vi "timeOfDayFromSS1904.vi"() -> (0 "New Values In":string[][](array[string])=[["Test data5"]], 1 "New Chs In":string[](array[string])=["30-10-03:New:Channel new5"])   [LabVIEW 2022 SP3]
uses:
  Data plotting/subVIs/Plot_Values_Global.vi
panel:
  # "Using SS1/1/1904 on the X-axis, adds channels for Hour and Minute"
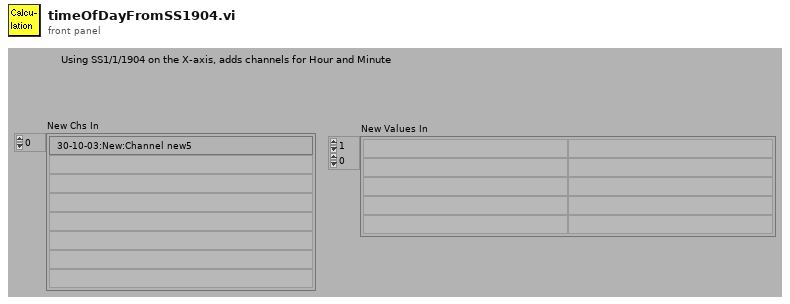
[diagram p1: front panel]
types:
  T1 = typedef "LVDateTimeRec.ctl" = cluster{"fractional second":dbl, "second":i32, "minute":i32, "hour":i32, "day of month":i32, "month":i32, "year":i32, "day of week":i32, "day of year":i32, "DST":i32}
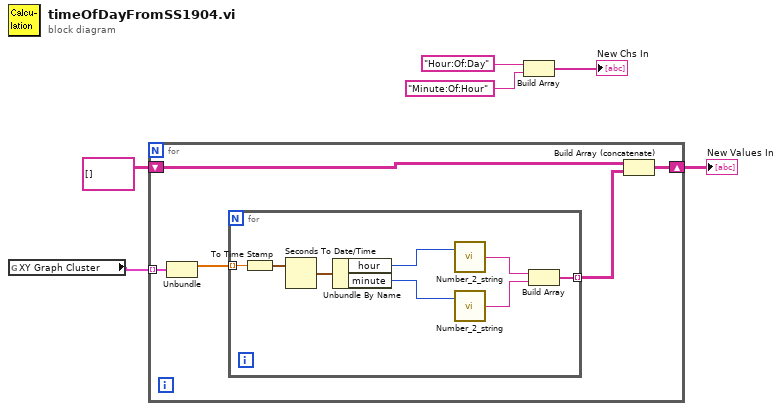
[diagram p0: block diagram]
diagram:
  n1 = global read "Plot_Values_Global.vi" "XY Graph Cluster"() -> (w2:cluster{dbl[], dbl[]}[])
  n2 = for {
    tunnel: w2 -> [w11] mode=indexing
    shift-right: [w9] -> w4
    shift-left: string[][] [] -> [w10]
    n3 = Unbundle(w11) -> (w7:dbl[])  [unwired: 1 out]
    n4 = for {
      tunnel: w7 -> [w17] mode=indexing
      tunnel: [w18] -> w8 mode=indexing
      n5 = To Time Stamp(1:w17) -> (0:w16:timestamp)
      n6 = Seconds To Date/Time(time stamp (now)=w16) -> (date time rec=w15:T1)  [unwired: 1 in]
      n7 = Unbundle By Name(w15) -> ("hour"=w14:i32, "minute"=w13:i32)
      n8 = call "Number_2_string.vi"("number"=w14) -> ("String"=w19:string)  [unwired: 1 in]
      n9 = call "Number_2_string.vi"("number"=w13) -> ("String"=w12:string)  [unwired: 1 in]
      n10 = Build Array(w19, w12) -> (w18:string[])
    }
    n11 = Build Array (concatenate)(w10, w8) -> (w9:string[][])
  }
  "New Values In" <- w4
  n12 = Build Array("Hour:Of:Day" ("string"), "Minute:Of:Hour" ("string")) -> (→"New Chs In":string[])
